vi "Scale Teaching Validation Vector.vi"(9 "Output Scaling":T3, 10 "Input Scaling":T3, 11 "Teaching/Validation Vector In":T1[](array[typedef])) -> (3 "Scaled Teaching/Validation Vector Out":T1[](array[typedef]))   [LabVIEW 2013, in "Super Simple Neural Network.lvlib"]
uses:
  Super Simple Neural Network.lvlib
  Types/Scaling Info.ctl
  Types/Teaching Vector.ctl
  Types/1D Array.ctl
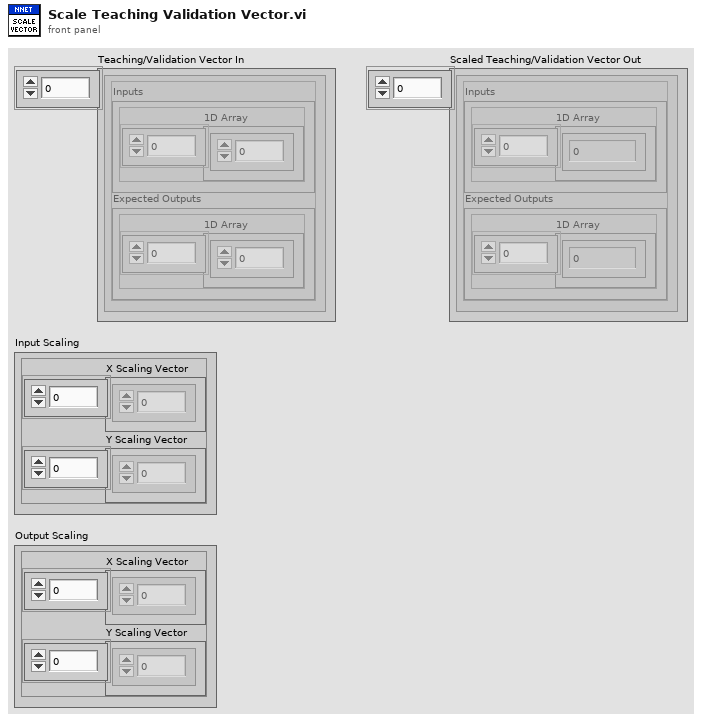
[diagram p1: front panel]
types:
  T1 = typedef "Super Simple Neural Network.lvlib/Teaching Vector.ctl" = cluster{"Inputs":T2, "Expected Outputs":T2}
  T2 = typedef "Super Simple Neural Network.lvlib/1D Array.ctl" = cluster{"1D Array":dbl[]}
  T3 = typedef "Super Simple Neural Network.lvlib/Scaling Info.ctl" = cluster{"X Scaling Vector":dbl[], "Y Scaling Vector":dbl[]}
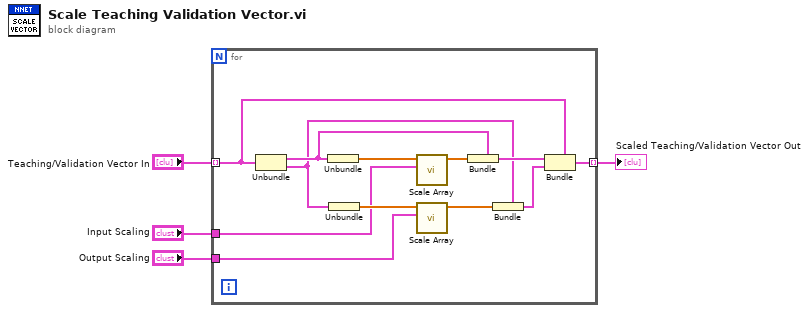
[diagram p0: block diagram]
diagram:
  n1 = for {
    tunnel: "Teaching/Validation Vector In" -> [w15] mode=indexing
    tunnel: [w7] -> w2 mode=indexing
    tunnel: "Input Scaling" -> [w6]
    tunnel: "Output Scaling" -> [w5]
    n2 = Unbundle(w15) -> ("Inputs"=w14:T2, "Expected Outputs"=w11:T2)
    n3 = Unbundle(w14) -> ("1D Array"=w16:dbl[])
    n4 = Unbundle(w11) -> ("1D Array"=w12:dbl[])
    n5 = call "Scale Array.vi"("Scaling Info"=w6, "Array to Scale"=w16) -> ("Scaled Array"=w9:dbl[])  [unwired: 9 in]
    n6 = call "Scale Array.vi"("Scaling Info"=w5, "Array to Scale"=w12) -> ("Scaled Array"=w10:dbl[])  [unwired: 9 in]
    n7 = Bundle(cluster=w14, "1D Array"=w9) -> (w13:T2)
    n8 = Bundle(cluster=w11, "1D Array"=w10) -> (w8:T2)
    n9 = Bundle(cluster=w15, "Inputs"=w13, "Expected Outputs"=w8) -> (w7:T1)
  }
  "Scaled Teaching/Validation Vector Out" <- w2
